vi "LSX Get V Level.vi"(7 "pdUppLevel":dbl, 8 "error in (no error)":errorcluster, 9 "pdDownLevel":dbl, 10 "lVRegion":i32, 11 "lLSID":i32) -> (0 "error out":errorcluster, 1 "pdDownLevel out":dbl, 3 "function return":i32, 5 "pdUppLevel out":dbl)   [LabVIEW 2018, in "Tango.lvlib"]
doc: "TANGOAPI int TANGOCALL LSX_GetVLevel (int lLSID, int lVRegion, double *pdDownLevel, double *pdUppLevel);"
uses:
  Tango.lvlib
  SubVIs/Tango_DLL.dll
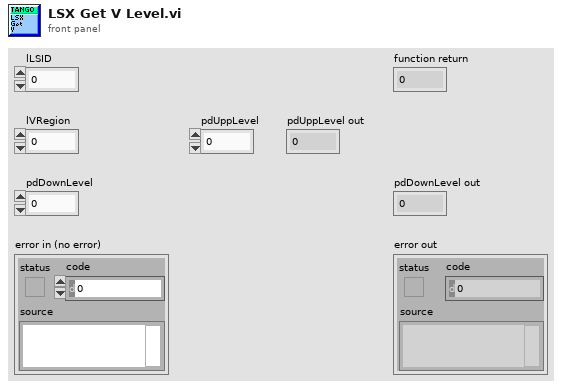
[diagram p1: front panel]
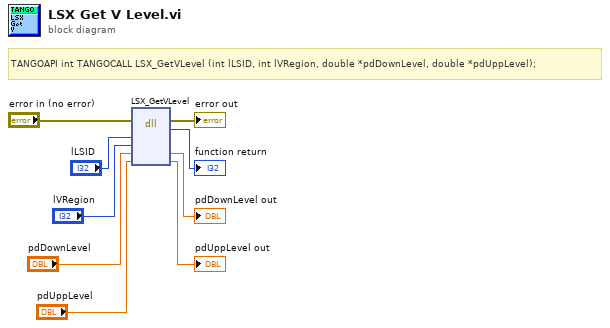
[diagram p0: block diagram]
diagram:
  # "TANGOAPI int TANGOCALL LSX_GetVLevel (int lLSID, int lVRegion, double *pdDownLevel, double *pdUppLevel);"
  n1 = dll-call lib="C:/Users/Familie/Documents/LabviewIX81/lib/TANGO Stage/SubVIs/Tango_DLL.*" fn="LSX_GetVLevel"(error in="error in (no error)", "lLSID"="lLSID", "lVRegion"="lVRegion", "pdDownLevel"="pdDownLevel", "pdUppLevel"="pdUppLevel") -> (error out=→"error out":errorcluster, →"function return":i32, "pdDownLevel"=→"pdDownLevel out":dbl, "pdUppLevel"=→"pdUppLevel out":dbl)  [unwired: 4 in, 1 out]
